vi "Photo Current Calculator (SubVI).vi"(10 "G (w/m^2)":dbl, 11 "T (K)":dbl) -> (3 "I_ph":dbl)   [LabVIEW 2024]
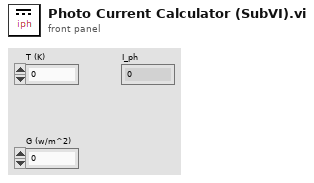
[diagram p1: front panel]
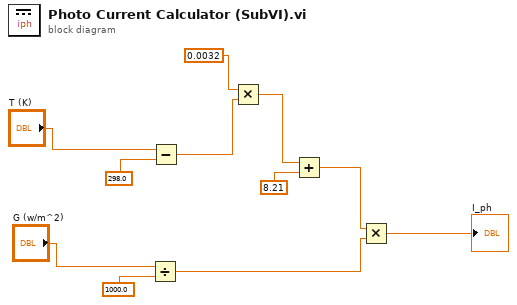
[diagram p0: block diagram]
diagram:
  n1 = Divide(x="G (w/m^2)", y=1000.0) -> (x/y=w7:dbl)
  n2 = Subtract(x="T (K)", y=298.0) -> (x-y=w5:dbl)
  n3 = Multiply(x=0.0032, y=w5) -> (x*y=w6:dbl)
  n4 = Add(x=w6, y=8.21) -> (x+y=w9:dbl)
  n5 = Multiply(x=w9, y=w7) -> (x*y=→"I_ph":dbl)
